vi "Ex4-get-data.vi"() -> ()   [LabVIEW 2021]
uses:
  <vilib>/Utility/NIReport.llb/Report Type.ctl
  <vilib>/addons/_office/excel.llb/Excel Get Data ([dbl]).vi
  <vilib>/Utility/NIReport.llb/NI_report.lvclass
  <vilib>/Utility/NIReport.llb/NI_ReportGenerationCore.lvlib
  <vilib>/Utility/NIReport.llb/Excel/NI_Excel.lvclass
  <vilib>/addons/_office/NI_ReportGenerationToolkit.lvlib
  <vilib>/addons/_office/excel.llb/Excel Easy Table (str).vi
panel:
  out "data":dbl[][](array[numeric]) format="%.2f"
  out "size(s)":i32[](array[numeric])
  in  "stop":bool
  out "MS Office parameters out":T1
  in  "Text Ring":u16(ring) items=["data1", "data2", "data3", "data4", "data5", "summary"]
  out "Work sheet names":string[](array[string])
  out "Count":i32
  in  "file path (use dialog)":path
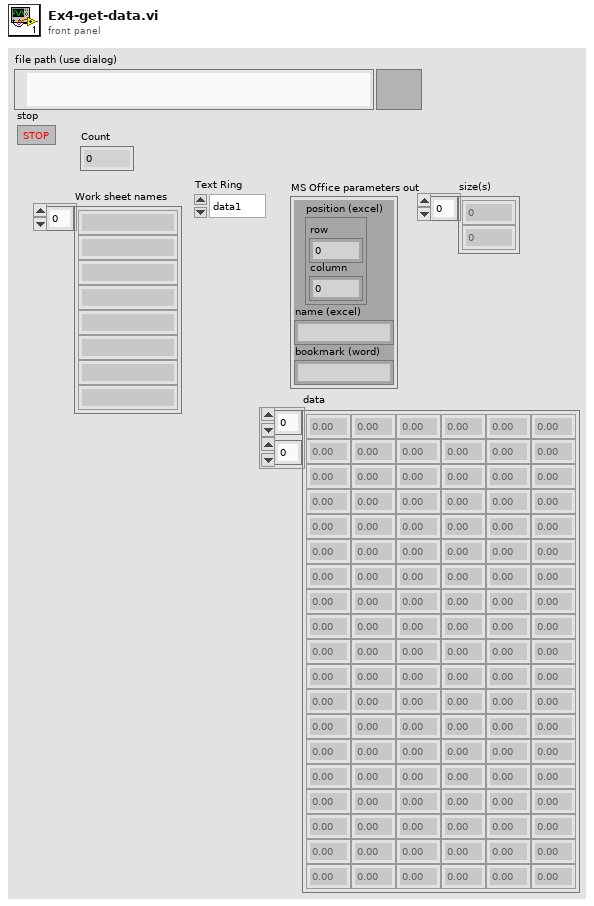
[diagram p1: front panel]
types:
  T1 = cluster{"position (excel)":cluster{"row":i32, "column":i32}, "name (excel)":string, "bookmark (word)":string}
  T2 = enum16{"open", "replace", "create", "open or create", "replace or create", "replace or create with confirmation"}
  T3 = typedef "NI_ReportGenerationCore.lvlib/Report Type.ctl" = enum16{"HTML", "Word", "Excel"}
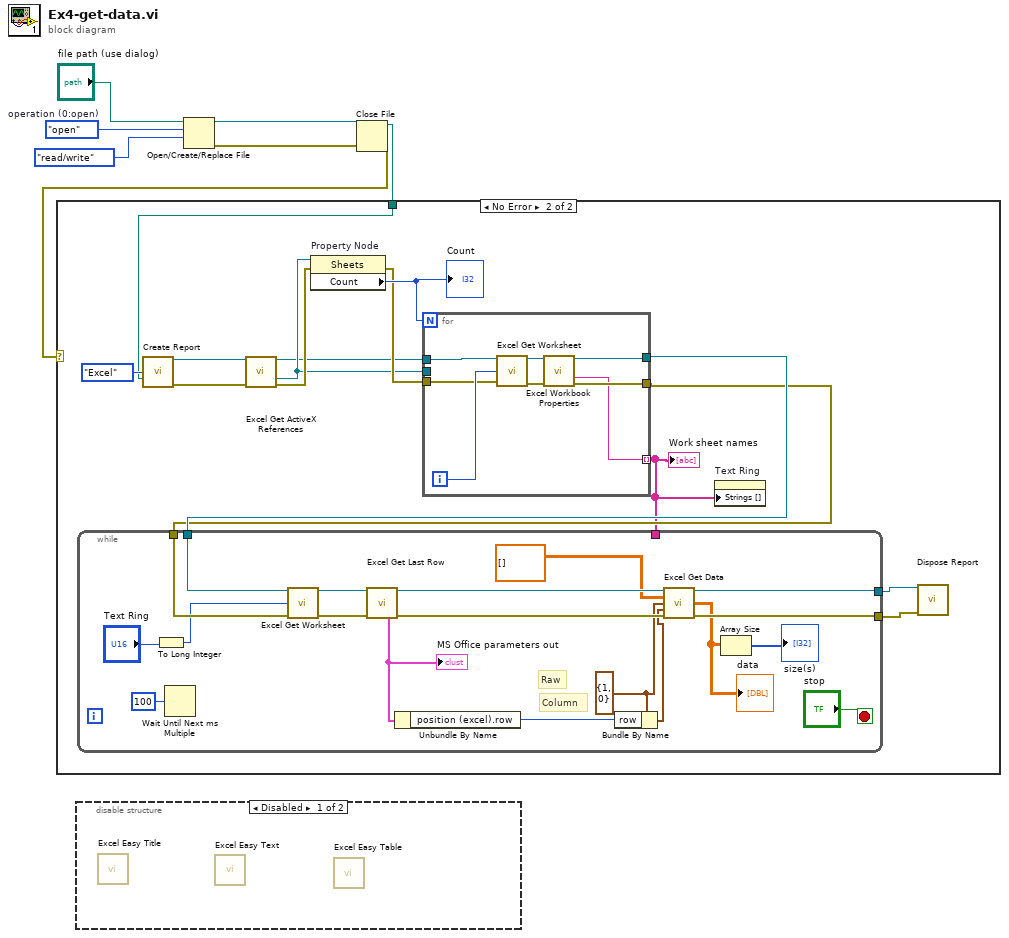
[diagram p0: block diagram]
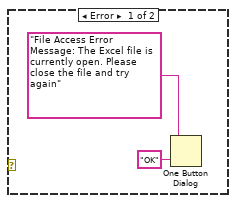
[diagram p3: hidden frame]
diagram:
  w4 = T2."open"  # operation (0:open)
  n1 = disable-structure shown="Disabled" {
    frame Disabled {
      n2 = call <vilib>:"Excel Easy Title.vi"() -> ()  [unwired: 13 in, 3 out]
      n3 = call <vilib>:"Excel Easy Text.vi"() -> ()  [unwired: 11 in, 5 out]
      n4 = call-poly <vilib>:"Excel Easy Table.vi"() -> ()  [unwired: 11 in, 5 out]
    }
    frame Enabled {
    }
  }
  n5 = Open/Create/Replace File(file path (use dialog)="file path (use dialog)", operation (0:open)=w4, access (0:read/write)=enum16{"read/write", "read-only", "write-only"}."read/write") -> (refnum out=w7:refnum<file>, error out=w6:errorcluster)  [unwired: 3 in, 1 out]
  n6 = Close File(refnum=w7, error in=w6) -> (path=w1:path, error out=w2:errorcluster)
  n7 = case shown="No Error" w2 {
    tunnel: w1 -> [_ w22]
    frame Error {
      n8 = One Button Dialog(message="File Access Error Message: The Excel file is currently open. Please close the file and try again", button name ("OK")="OK") -> ()  [unwired: 1 out]
    }
    frame No Error {
      n9 = call <vilib>:"Create Report.vi"("report type"=Report_Type."Excel", "template (empty)"=w22) -> ("report out"=w21:refnum<class "NI_report.lvclass">, "error out"=w20:errorcluster)  [unwired: 12 in]
      n10 = call <vilib>:"Excel Get ActiveX References.vi"("report in"=w21, "error in (no error)"=w20) -> ("report out"=w15:refnum<class "NI_report.lvclass">, "Excel.Sheets"=w16:refnum<k7>, "error out"=w18:errorcluster)  [unwired: 7 in, 4 out]
      n11 = property on="Property Node" class="Sheets"(reference=w16, error in=w18) -> (error out=w17:errorcluster, "Count"=w19:i32)  [unwired: 1 out]
      "Count" <- w19
      n12 = for {
        N: w19 -> [_]
        tunnel: w17 -> [w44]
        tunnel: w16 -> [_]
        tunnel: w15 -> [w49]
        tunnel: [w47] -> w14
        tunnel: [w45] -> w13
        tunnel: [w43] -> w12 mode=indexing
        i -> [w50]
        n13 = call <vilib>:"Excel Get Worksheet.vi"("report in"=w49, "worksheet index (0)"=w50, "error in (no error)"=w44) -> ("report out"=w48:refnum<class "NI_report.lvclass">, "error out"=w46:errorcluster)  [unwired: 11 in]
        n14 = call <vilib>:"Excel Workbook Properties.vi"("report in"=w48, "error in (no error)"=w46) -> ("report out"=w47:refnum<class "NI_report.lvclass">, "current worksheet name"=w43:string, "error out"=w45:errorcluster)  [unwired: 10 in, 1 out]
      }
      "Work sheet names" <- w12
      n15 = while {
        tunnel: w12 -> [_]
        tunnel: w14 -> [w42]
        tunnel: w13 -> [w41]
        tunnel: [w31] -> w11
        tunnel: [w30] -> w10
        stop <- "stop" stop-if-true
        w27 = cluster{"row":i32, "column":i32} {"row"=1, "column"=0} ("start (-1, -1)")
        # "Raw"
        # "Column"
        n16 = To Long Integer(number="Text Ring") -> (32bit integer=w39:i32)
        n17 = Wait Until Next ms Multiple(millisecond multiple=u32 100) -> ()  [unwired: 1 out]
        n18 = call <vilib>:"Excel Get Worksheet.vi"("report in"=w42, "worksheet index (0)"=w39, "error in (no error)"=w41) -> ("report out"=w38:refnum<class "NI_report.lvclass">, "error out"=w37:errorcluster)  [unwired: 11 in]
        n19 = call <vilib>:"Excel Get Last Row.vi"("report in"=w38, "error in (no error)"=w37) -> ("report out"=w34:refnum<class "NI_report.lvclass">, "MS Office parameters out"=w26:T1, "error out"=w32:errorcluster)  [unwired: 11 in]
        "MS Office parameters out" <- w26
        n20 = Unbundle By Name(w26) -> ("position (excel).row"=w25:i32)
        n21 = Bundle By Name(cluster=w27, "row"=w25) -> (w24:cluster{"row":i32, "column":i32})
        n22 = call-poly <vilib>:"Excel Get Data.vi"("report in"=w34, "data type"=dbl[][] [], "start (-1, -1)"=w27, "end (-1, -1)"=w24, "error in (no error)"=w32) -> ("report out"=w31:refnum<class "NI_report.lvclass">, "data"=w29:dbl[][], "error out"=w30:errorcluster)  [unwired: 8 in]
        "data" <- w29
        n23 = Array Size(array=w29) -> (size(s)=→"size(s)":i32[])
      }
      n24 = property on="Text Ring" class="Ring (strict)"("Strings []"=w12) -> ()  [unwired: 2 in, 2 out]
      n25 = call-dynamic "Dispose Report.vi"("report in"=w11, "error in (no error)"=w10) -> ()  [unwired: 13 in, 1 out]
    }
  }
